vi "FG_ICON Data from Tag.vi"(8 "Error":errorcluster, 10 "Default Body Text":T3 {"Body Text Spec"."Alignment" items=["left", "center", "right"]}, 11 "Init? (F)":bool) -> (0 "Error Out":errorcluster, 1 "Library Icon Out":picture, 2 "Invoked Data Out":T1, 3 "Data Out":T6={"Text Visible?"=FALSE, "Text Opacity"=0, "Templ Visible?"=FALSE, "Templ Opacity"=0, "Relative Path from 1 to 2"=path "", "Image"=bytes[0], "All User Layers"=[], "Body Text"={"Line 1 text"="", "Line 2 text"="", "Line 3 text"="", "Line 4 text"="", "Line 1 color"=0, "Line 2 color"=0, "Line 3 color"=0, "Line 4 color"=0, "Body Text Spec"={"Font"="", "Alignment"=0, "Size"=3}, "Center text vertically"=FALSE, "Capitalize Text"=FALSE}} {"Body Text"."Body Text Spec"."Alignment" items=["left", "center", "right"]}, 4 "Valid? Out":bool, 5 "Valid Library Icon? Out":bool)   [LabVIEW 2021]
uses:
  vi.lib/LabVIEW Icon API/lv_icon/Controls/LabVIEW Icon Stored Information.ctl
  vi.lib/LabVIEW Icon API/lv_icon/Classes/Layer/Layer.lvclass
  TypeDefs/Cluster_BodyText.ctl
  vi.lib/LabVIEW Icon API/lv_icon/Controls/Font.ctl
  vi.lib/LabVIEW Icon API/lv_icon/Controls/Alignment.ctl
  <resource>/plugins/IconEditor/Who Invoked Icon Editor.ctl
  <resource>/plugins/IconEditor/Icon Editor Invoker Type.ctl
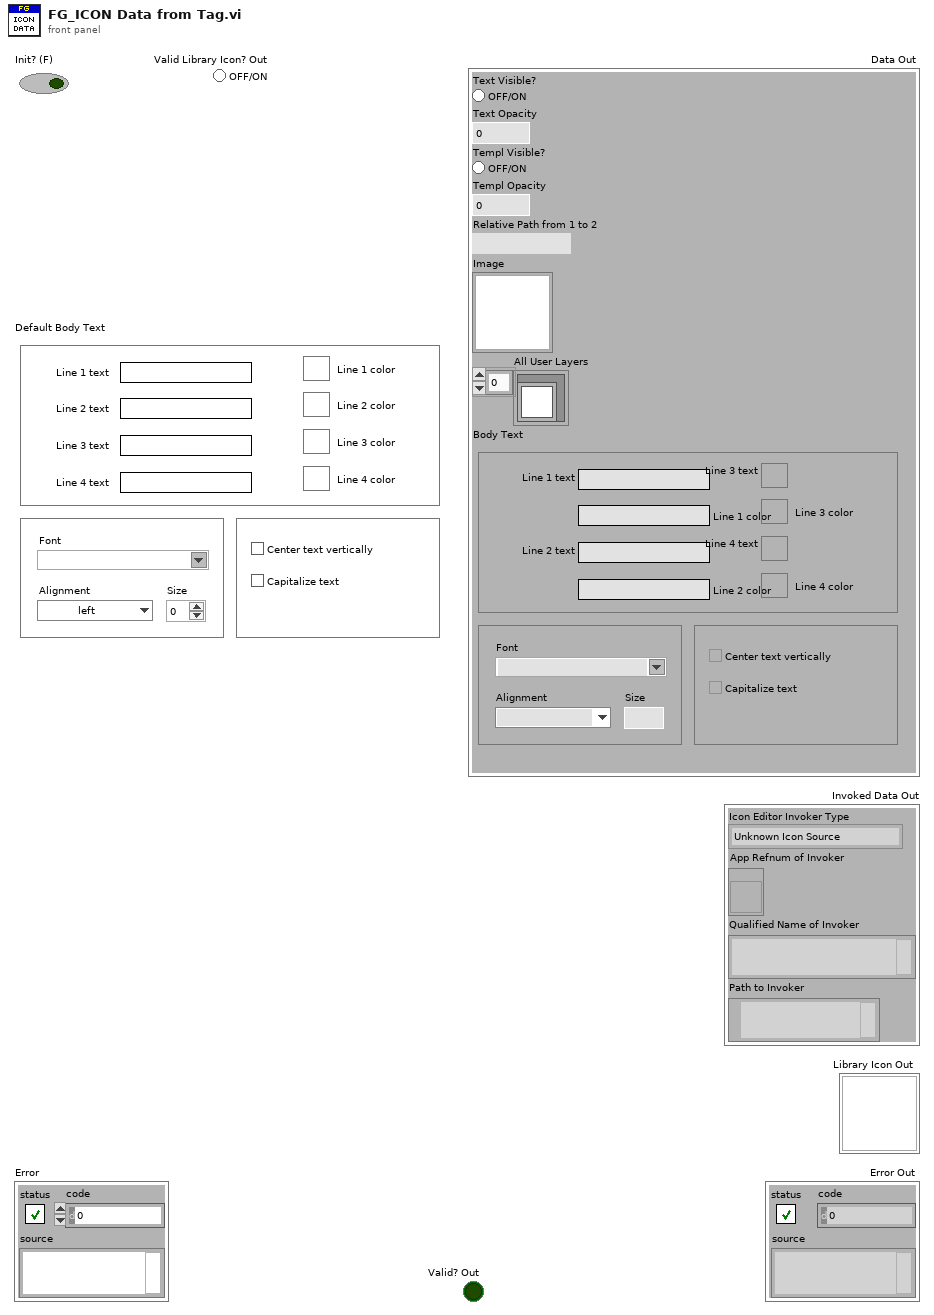
[diagram p1: front panel]
types:
  T1 = typedef "Who Invoked Icon Editor.ctl" = cluster{"Icon Editor Invoker Type":T2, "App Refnum of Invoker":refnum<vi>, "Qualified Name of Invoker":string, "Path to Invoker":path}
  T2 = typedef "Icon Editor Invoker Type.ctl" = enum32{"Unknown Icon Source", "VI Icon", "Library Icon (any library type)", "Palette icon", "Icon from App Method"}
  T3 = typedef "Cluster_BodyText.ctl" = cluster{"Line 1 text":string, "Line 2 text":string, "Line 3 text":string, "Line 4 text":string, "Line 1 color":u32, "Line 2 color":u32, "Line 3 color":u32, "Line 4 color":u32, "Body Text Spec":cluster{"Font":T4, "Alignment":T5, "Size":u8}, "Center text vertically":bool, "Capitalize Text":bool}
  T4 = typedef "Font.ctl" = string
  T5 = typedef "Alignment.ctl" = u16
  T6 = typedef "LabVIEW Icon Stored Information.ctl" = cluster{"Text Visible?":bool, "Text Opacity":u8, "Templ Visible?":bool, "Templ Opacity":u8, "Relative Path from 1 to 2":path, "Image":picture, "All User Layers":refnum<class "Layer.lvclass">[], "Body Text":T3}
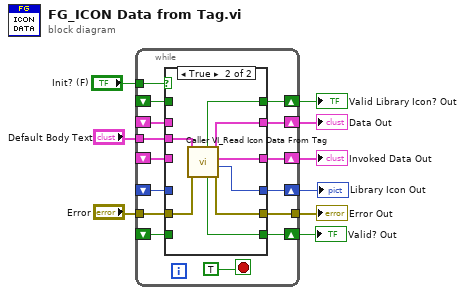
[diagram p0: block diagram]
diagram:
  n1 = while {
    tunnel: [w24] -> w9
    tunnel: "Error" -> [w21]
    tunnel: "Init? (F)" -> [w20]
    shift-right: [w22] -> w5
    shift-left: _ -> [w18]
    shift-right: [w23] -> w6
    shift-left: _ -> [w17]
    shift-right: [w16] -> w4
    shift-left: _ -> [w15]
    shift-right: [w14] -> w3
    shift-left: _ -> [w13]
    tunnel: "Default Body Text" -> [w12]
    shift-right: [w11] -> w1
    shift-left: _ -> [w10]
    stop <- TRUE stop-if-true
    n2 = case shown="True" w20 {
      tunnel: [w28 w38] -> w24
      tunnel: [w30 w37] -> w22
      tunnel: [w29 w36] -> w23
      tunnel: w21 -> [w28 w35]
      tunnel: w18 -> [w30 _]
      tunnel: w17 -> [w29 _]
      tunnel: [w27 w34] -> w16
      tunnel: w15 -> [w27 _]
      tunnel: [w26 w32] -> w14
      tunnel: w13 -> [w26 _]
      tunnel: w12 -> [_ w33]
      tunnel: [w25 w31] -> w11
      tunnel: w10 -> [w25 _]
      frame False {
      }
      frame True {
        n3 = call "Caller VI_Read Icon Data From Tag.vi"("Error"=w35, "Default Body Text"=w33) -> ("Error Out"=w38:errorcluster, "Library Icon If Valid"=w34:picture, "Who Invoked The Icon Editor? Out"=w31:T1, "Data Out"=w37:T6, "Valid? Out"=w36:bool, "Valid Library Icon? Out"=w32:bool)  [unwired: 4 in]
      }
    }
  }
  "Error Out" <- w9
  "Valid? Out" <- w6
  "Data Out" <- w5
  "Library Icon Out" <- w4
  "Valid Library Icon? Out" <- w3
  "Invoked Data Out" <- w1
